vi "Get Errno.vi"(8 "error in (no error)":errorcluster) -> (0 "error out":errorcluster, 3 "errno":u32)   [LabVIEW 2017, in "Utilities.lvlib"]
doc: "Gets errno for the current thread.\nResets the errno if called."
uses:
  Utilities.lvlib
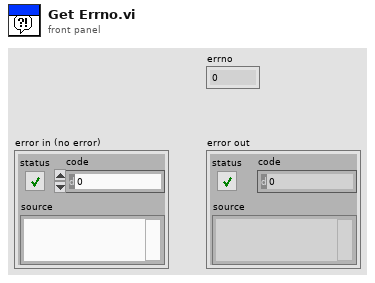
[diagram p1: front panel]
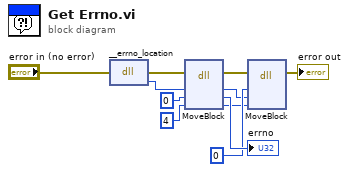
[diagram p0: block diagram]
diagram:
  n1 = dll-call lib="LabVIEW" fn="__errno_location"(error in="error in (no error)") -> (error out=w11:errorcluster, "return type"=w6:u64)  [unwired: 2 in, 1 out]
  n2 = dll-call lib="LabVIEW" fn="MoveBlock"(error in=w11, "pointer"=w6, "data"=u32 0 ("size"), "size"=u64 4) -> (error out=w2:errorcluster, "pointer"=w3:u64, "data"=→"errno":u32, "size"=w4:u64)  [unwired: 3 in, 1 out]
  n3 = dll-call lib="LabVIEW" fn="MoveBlock"(error in=w2, "data"=u32 0 ("size"), "pointer"=w3, "size"=w4) -> (error out=→"error out":errorcluster)  [unwired: 6 in, 1 out]
